vi "Timer Temparature.vi"(8 "error in":errorcluster, 9 "Refresh Time":dbl, 10 "Set Time":dbl, 11 "Options":T1) -> (0 "error out":errorcluster, 1 "Elapsed time":dbl, 2 "Refresh?":bool, 3 "Timeout?":bool)   [LabVIEW 2023, in "LTT_TeststandSteptypes.lvlib"]
uses:
  LTT_TeststandSteptypes.lvlib
  HardwareAbstractionLayer_LVOOP/Power Moniter/Wait Monitor_class/SubVI/Control/TimerStates.ctl
  HardwareAbstractionLayer_LVOOP/Power Moniter/Wait Monitor_class/Wait Monitor.lvclass
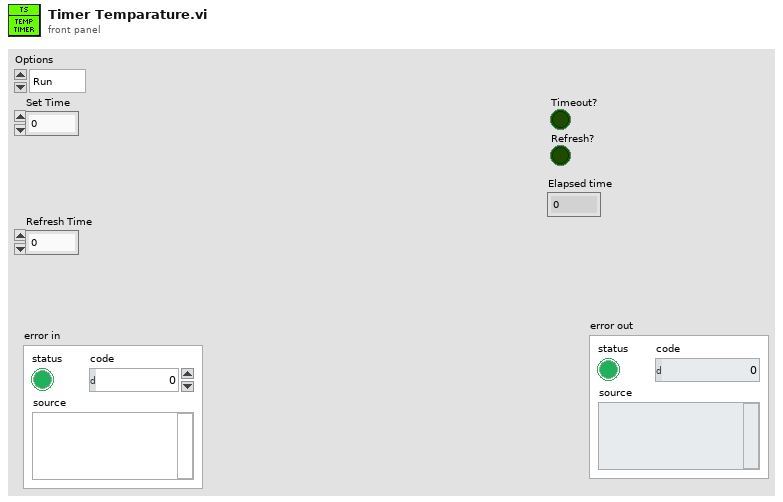
[diagram p1: front panel]
types:
  T1 = typedef "HardwareAbstractionLayer_LVOOP.lvlib/Wait Monitor.lvclass/TimerStates.ctl" = enum16{"Run", "Pause", "Reset"}
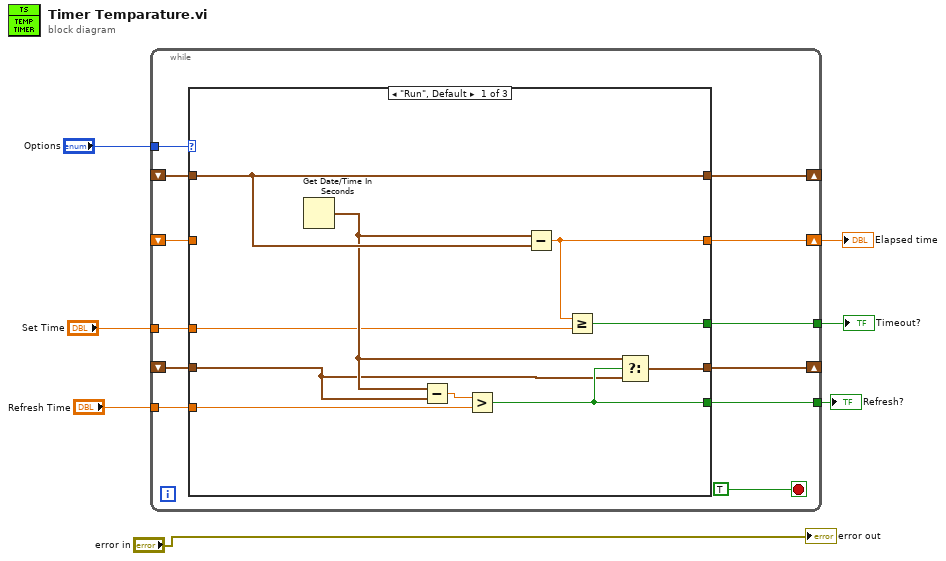
[diagram p0: block diagram]
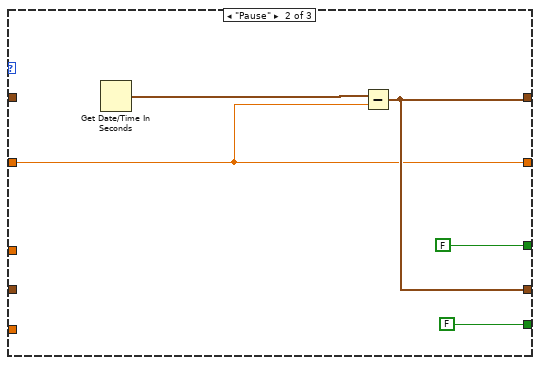
[diagram p2: hidden frame]
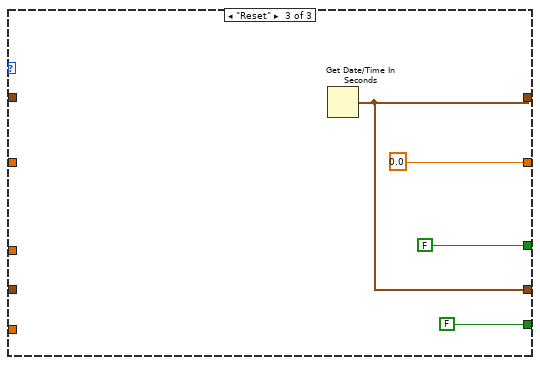
[diagram p3: hidden frame]
diagram:
  n1 = while {
    tunnel: "Options" -> [w19]
    shift-right: [w16] -> _
    shift-left: _ -> [w17]
    tunnel: "Set Time" -> [w15]
    tunnel: [w13] -> w4
    shift-right: [w14] -> w5
    shift-left: _ -> [w12]
    tunnel: "Refresh Time" -> [w11]
    tunnel: [w10] -> w1
    shift-right: [w9] -> _
    shift-left: _ -> [w8]
    stop <- TRUE stop-if-true
    n2 = case shown="\"Run\", Default" w19 {
      tunnel: [w20 w30 0.0] -> w14
      tunnel: w17 -> [w29 _ _]
      tunnel: [w29 w31 w36] -> w16
      tunnel: [w28 FALSE FALSE] -> w13
      tunnel: w15 -> [w21 _ _]
      tunnel: w12 -> [_ w30 _]
      tunnel: w11 -> [w27 _ _]
      tunnel: [w26 FALSE FALSE] -> w10
      tunnel: [w25 w31 w36] -> w9
      tunnel: w8 -> [w22 _ _]
      frame "Run", Default {
        n3 = Get Date/Time In Seconds() -> (seconds since 1Jan1904=w24:timestamp)
        n4 = Subtract(x=w24, y=w22) -> (x-y=w23:dbl)
        n5 = Greater?(x=w23, y=w27) -> (0:w26:bool)
        n6 = Subtract(x=w24, y=w29) -> (x-y=w20:dbl)
        n7 = Greater Or Equal?(x=w20, y=w21) -> (x >= y?=w28:bool)
        n8 = Select(t=w24, s=w26, f=w22) -> (s? t:f=w25:timestamp)
      }
      frame "Pause" {
        n9 = Get Date/Time In Seconds() -> (seconds since 1Jan1904=w32:timestamp)
        n10 = Subtract(x=w32, y=w30) -> (x-y=w31:timestamp)
      }
      frame "Reset" {
        n11 = Get Date/Time In Seconds() -> (seconds since 1Jan1904=w36:timestamp)
      }
    }
  }
  "Elapsed time" <- w5
  "Timeout?" <- w4
  "Refresh?" <- w1
  "error out" <- "error in"
